vi "get_GPIB_settings.vi"(8 "error in (no error)":errorcluster, 11 "config_file_name":string="VISA_config.ini") -> (0 "error out":errorcluster, 2 "GPIB settings":T1, 3 "config_file_name_out":string)   [LabVIEW 2015]
uses:
  <vilib>/Utility/config.llb/Read Key (String).vi
  <vilib>/Utility/config.llb/NI_LVConfig.lvlib
panel:
  # "Devuelve las direcciones de los puertos GPIB del archivo de configuración"
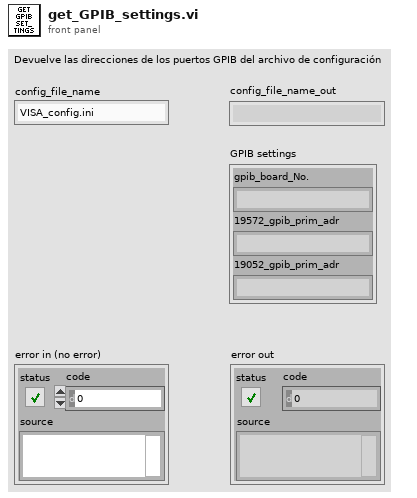
[diagram p1: front panel]
types:
  T1 = cluster{"gpib_board_No.":string, "19572_gpib_prim_adr":string, "19052_gpib_prim_adr":string}
  T2 = cluster{"[0]":string, "[1]":string, "[2]":string}
  T3 = typedef "NI_LVConfig.lvlib/Config Data RefNum.ctl" = refnum<k1>
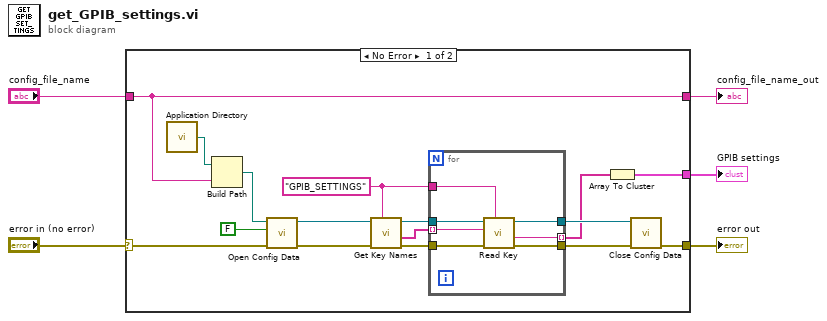
[diagram p0: block diagram]
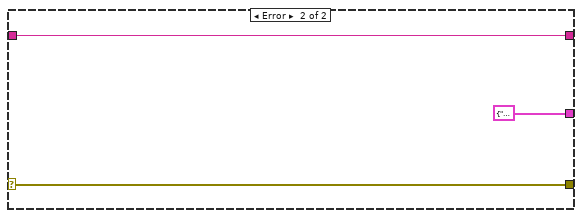
[diagram p2: hidden frame]
diagram:
  n1 = case shown="No Error" "error in (no error)" {
    selector: "error in (no error)" -> [w12 w31]
    tunnel: [w11 w31] -> w5
    tunnel: [w10 w30] -> w3
    tunnel: "config_file_name" -> [w10 w30]
    tunnel: [w6 T2 {"[0]"="", "[1]"="", "[2]"=""}] -> w1
    frame No Error {
      w17 = "GPIB_SETTINGS" ("section")
      n2 = call <vilib>:"Application Directory.vi"() -> ("Application Directory"=w19:path)
      n3 = Build Path(base path=w19, name or relative path=w10) -> (appended path=w18:path)
      n4 = call <vilib>:"Open Config Data.vi"("error in (no error)"=w12, "create file if necessary (T)"=FALSE, "configuration file path"=w18) -> ("error out"=w21:errorcluster, "refnum"=w20:T3)  [unwired: 6 in, 1 out]
      n5 = call <vilib>:"Get Key Names.vi"("section"=w17, "error in (no error)"=w21, "refnum"=w20) -> ("error out"=w15:errorcluster, "key names"=w9:string[], "refnum out"=w16:T3)  [unwired: 5 in, 1 out]
      n6 = for {
        tunnel: w9 -> [w28] mode=indexing
        tunnel: [w27] -> w7 mode=indexing
        tunnel: w17 -> [w26]
        tunnel: w16 -> [w25]
        tunnel: w15 -> [w24]
        tunnel: [w23] -> w14
        tunnel: [w22] -> w13
        n7 = call-poly <vilib>:"Read Key.vi"("section"=w26, "error in (no error)"=w24, "key"=w28, "refnum"=w25) -> ("error out"=w22:errorcluster, "value"=w27:string, "refnum out"=w23:T3)  [unwired: 4 in, 1 out]
      }
      n8 = Array To Cluster(array=w7) -> (cluster=w6:T2)
      n9 = call <vilib>:"Close Config Data.vi"("error in (no error)"=w13, "refnum"=w14) -> ("error out"=w11:errorcluster)  [unwired: 8 in, 1 out]
    }
    frame Error {
    }
  }
  "error out" <- w5
  "config_file_name_out" <- w3
  "GPIB settings" <- w1
